vi "CSMSVMgr Import Permanent Variable From File.vi"(8 "error in (no error)":errorcluster, 10 "Path":path, 11 "CSM-Static-Variable-Manager in":refnum<class "CSM-Static-Variable-Manager.lvclass">) -> (0 "error out":errorcluster, 3 "CSM-Static-Variable-Manager out":refnum<class "CSM-Static-Variable-Manager.lvclass">)   [LabVIEW 2017, in "INI-Static-Variable-Support.lvlib" / "CSM-Static-Variable-Manager.lvclass"]
uses:
  CSM-Static-Variable-Manager.lvclass
  CSM-Static-Variable-Manager.lvclass/CSM-Static-Variable-Manager.ctl
  LabVIEW-Config/LabVIEW-Config.lvlib
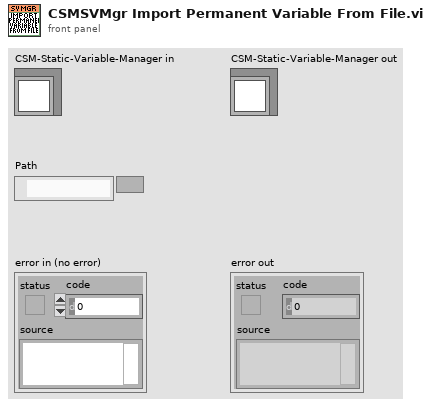
[diagram p1: front panel]
types:
  T1 = typedef "LabVIEW-Config.lvlib/Config.ctl" = cluster{"Path":path, "Lines":string[], "Tokens":enum8{"comment", "section", "key"}[], "Modified?":bool}
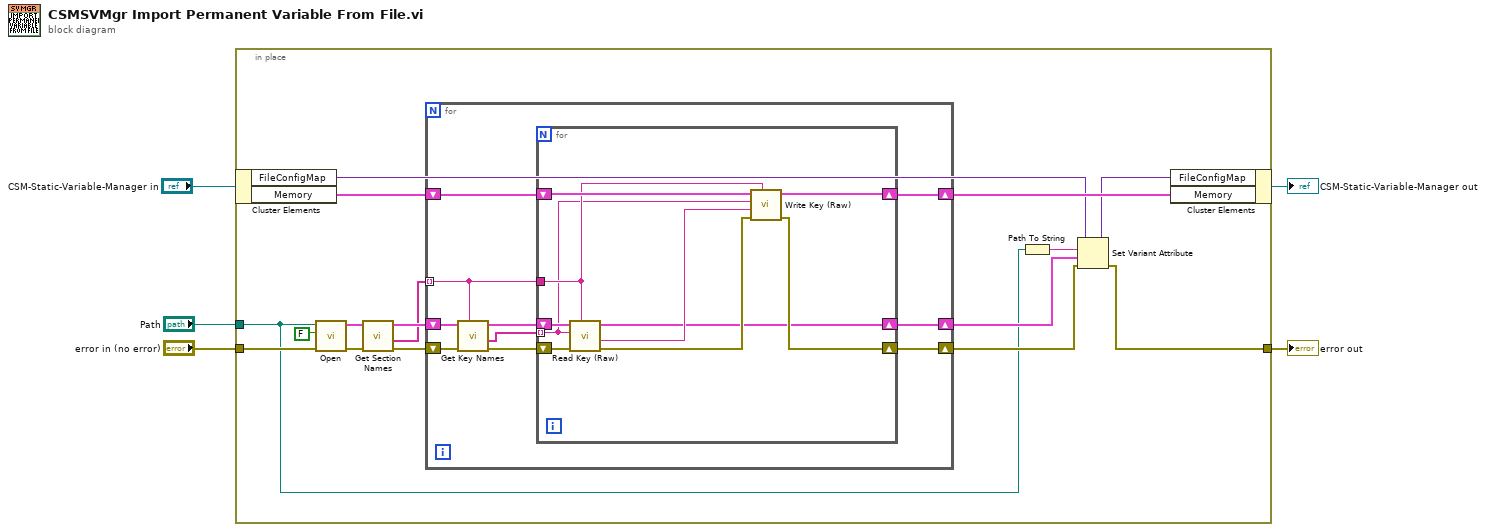
[diagram p0: block diagram]
diagram:
  n1 = in-place {
    in-place-border: "Path" -> [w7]
    in-place-border: "error in (no error)" -> [w11]
    in-place-border: [w8] -> w1
    n2 = in-place-cluster #1("CSM-Static-Variable-Manager in") -> ("FileConfigMap"=w13:variant, "Memory"=w15:T1)
    n3 = call "Open.vi"("error in (no error)"=w11, "Create if not exists? (T)"=FALSE, "Path"=w7) -> ("error out"=w20:errorcluster, "Config"=w19:T1)  [unwired: 5 in, 2 out]
    n4 = call "Get Section Names.vi"("error in (no error)"=w20, "Config in"=w19) -> ("error out"=w17:errorcluster, "Section Names"=w16:string[], "Config out"=w18:T1)  [unwired: 7 in]
    n5 = for {
      tunnel: w16 -> [w29] mode=indexing
      shift-right: [w24] -> w14
      shift-left: w15 -> [w25]
      shift-right: [w23] -> w9
      shift-left: w17 -> [w30]
      shift-right: [w22] -> w10
      shift-left: w18 -> [w31]
      n6 = call "Get Key Names.vi"("Section Name"=w29, "error in (no error)"=w30, "Config in"=w31) -> ("error out"=w26:errorcluster, "Key Names"=w27:string[], "Config out"=w28:T1)  [unwired: 5 in, 1 out]
      n7 = for {
        tunnel: w29 -> [w37]
        tunnel: w27 -> [w36] mode=indexing
        shift-right: [w33] -> w23
        shift-left: w26 -> [w40]
        shift-right: [w39] -> w24
        shift-left: w25 -> [w38]
        shift-right: [w32] -> w22
        shift-left: w28 -> [w41]
        n8 = call "Read Key (Raw).vi"("Section Name"=w37, "error in (no error)"=w40, "Key Name"=w36, "Config in"=w41) -> ("error out"=w34:errorcluster, "Content"=w35:string, "Config out"=w32:T1)  [unwired: 4 in, 1 out]
        n9 = call "Write Key (Raw).vi"("Section Name"=w37, "error in (no error)"=w34, "Content"=w35, "Key Name"=w36, "Config in"=w38) -> ("error out"=w33:errorcluster, "Config out"=w39:T1)  [unwired: 4 in, 1 out]
      }
    }
    n10 = Path To String(path=w7) -> (string=w6:string)
    n11 = Set Variant Attribute(Variant=w13, name=w6, value=w10, error in=w9) -> (Variant out=w12:variant, error out=w8:errorcluster)  [unwired: 1 out]
    n12 = in-place-cluster #1("FileConfigMap"=w12, "Memory"=w14) -> (→"CSM-Static-Variable-Manager out":refnum<class "CSM-Static-Variable-Manager.lvclass">)
  }
  "error out" <- w1
